vi "Main.vi"() -> ()   [LabVIEW 2020]
uses:
  Typedef/State.ctl
  Bundle Builder/Bundle Builder.lvclass
  Bundle Builder/Bundle Builder.lvclass/Bundle Builder.ctl
  bd79d48e-615b-41ab-9cb3-2d2f9496b7e1.vi
  Bundle Builder/Read Bundle Definition.vi
  Bundle Builder/Read Product Installers.vi
  Bundle Builder/Read Custom Actions.vi
  Bundle Builder/Read Element of Custom Actions Defnition.vi/bd8829dc-8fc1-4ce8-8fca-fa4916f1d24d.vi
  Bundle Builder/Read Element of Product Installers Definition.vi/92f76918-1563-4c6f-99b4-6a0cba476cd6.vi
  <vilib>/Comparison/Equal/Equal Functor/Equal Functor.lvclass
panel:
  in  "Clear Disk":bool
  in  "Stop Button":bool
  in  "Save":bool
  in  "Tab":T1(tab)
  in  "Bundle Definition":T2
  out "Product Key Unique?":bool
  in  "Product Installers":cluster{"Key":string, "Version":string}[](array[cluster])
  in  "Product Installer":T3 caption="NI Product Installer / Custom Product Installer"
  in  "Custom Actions":cluster{"Key":string, "Timing":string}[](array[cluster])
  out "Custom Action Key Unique?":bool
  in  "Custom Action":T4
  in  "Open":bool
  in  "Definitions":string(tree)
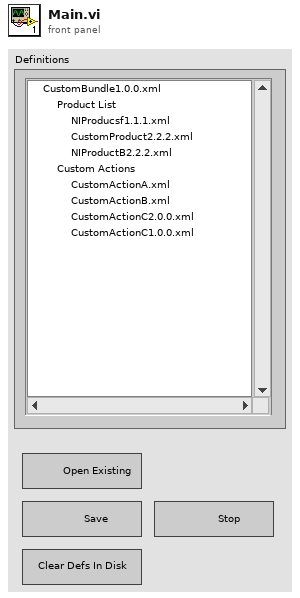
[diagram p1: front panel]
types:
  T1 = enum32{"Default", "Bundle", "Product List", "Product", "Custom Actions", "Custom Action"}
  T2 = cluster{"Key":string, "Display Name":string, "STS Software":string}
  T3 = cluster{"Display Name":string, "Type":enum16{"NI Installer", "Custom Installer"}, "Install Commands":cluster{"Path":string, "Parameters":string, "Successful Exit Codes":string, "Log Command":cluster{"Flag":string, "File Name":string}}[], "Uninstall Commands":cluster{"Path":string, "Parameters":string, "Successful Exit Codes":string, "Log Command":cluster{"Flag":string, "File Name":string}}[]}
  T4 = cluster{"Display Name":string, "Commands":cluster{"Path":string, "Parameters":string, "Successful Exit Codes":string}[]}
  T5 = typedef "State.ctl" = enum16{"Initialize", "Ready", "Open Bundle", "Show Selection Details"}
  T6 = enum8{"Enabled", "Disabled", "Disabled and Grayed Out"}
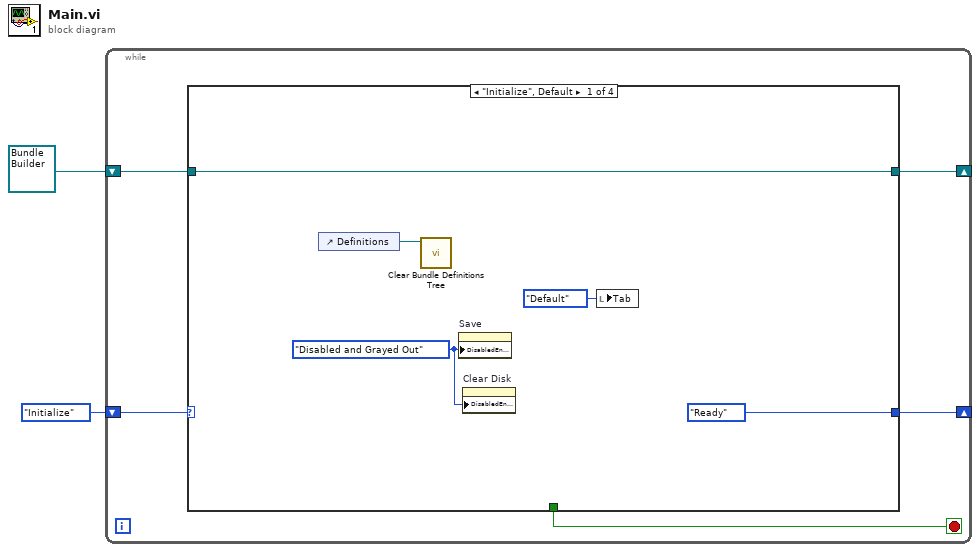
[diagram p0: block diagram]
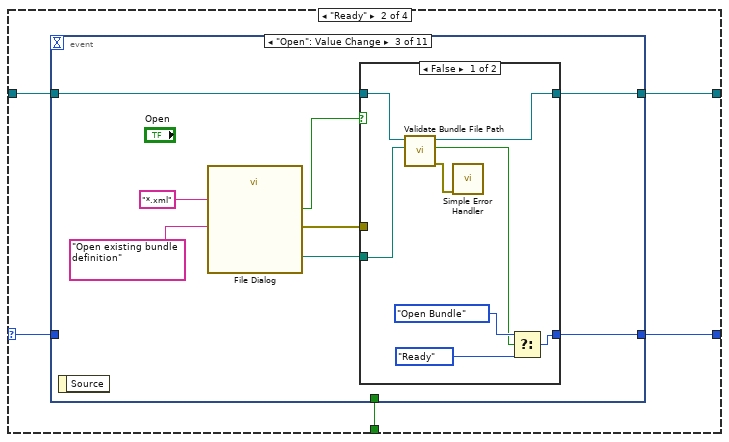
[diagram p2: hidden frame]
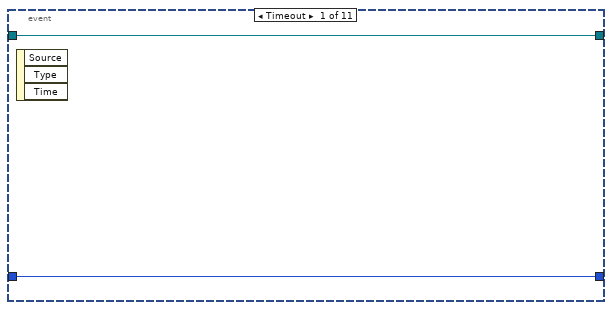
[diagram p3: hidden frame]
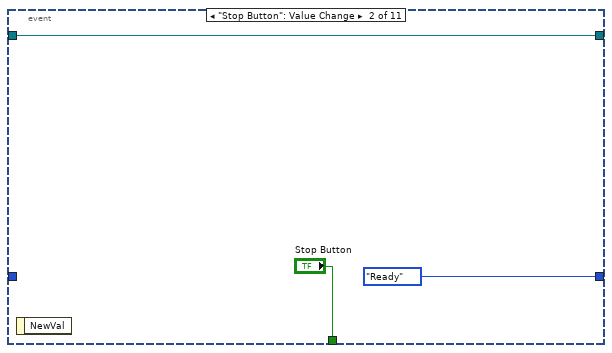
[diagram p4: hidden frame]
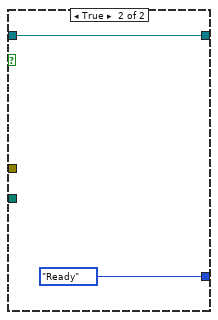
[diagram p5: hidden frame]
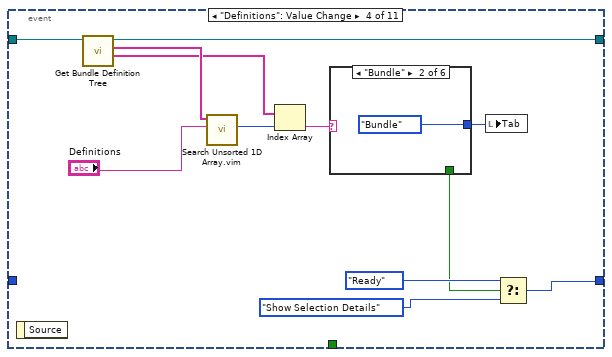
[diagram p6: hidden frame]
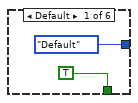
[diagram p7: hidden frame]
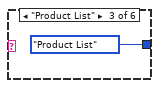
[diagram p8: hidden frame]
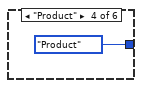
[diagram p9: hidden frame]
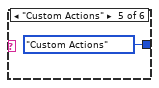
[diagram p10: hidden frame]
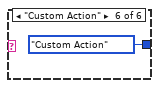
[diagram p11: hidden frame]
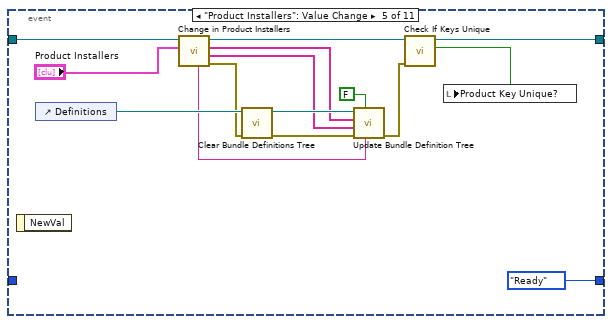
[diagram p12: hidden frame]
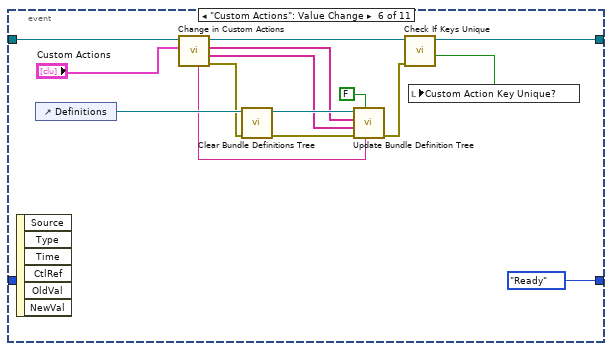
[diagram p13: hidden frame]
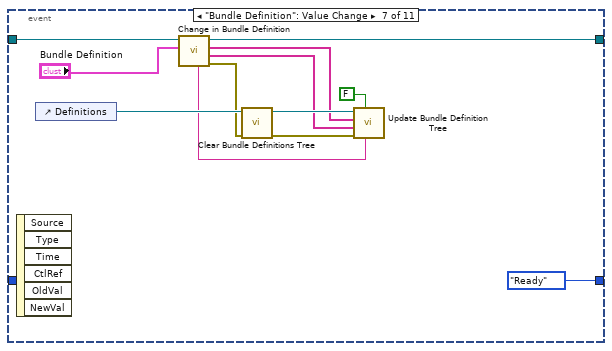
[diagram p14: hidden frame]
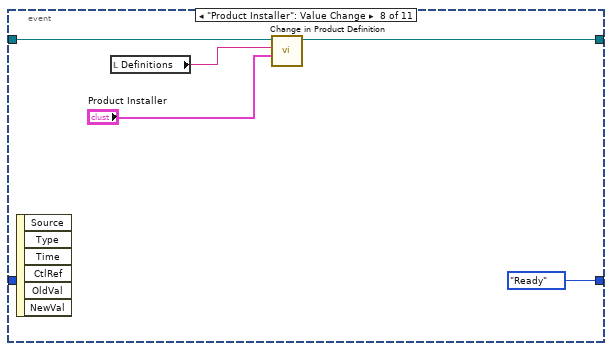
[diagram p15: hidden frame]
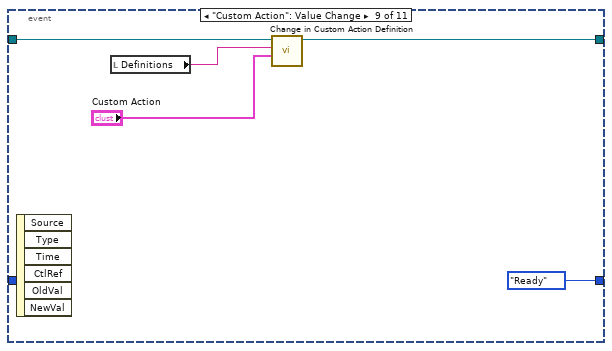
[diagram p16: hidden frame]
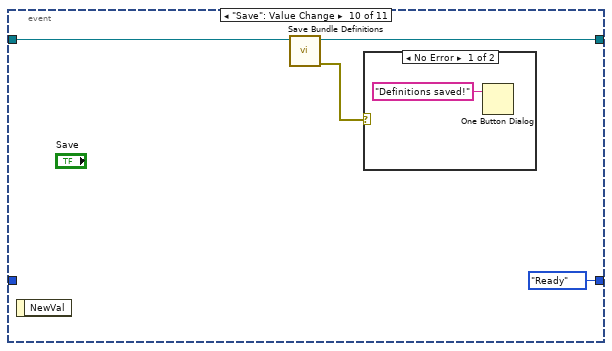
[diagram p17: hidden frame]
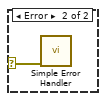
[diagram p18: hidden frame]
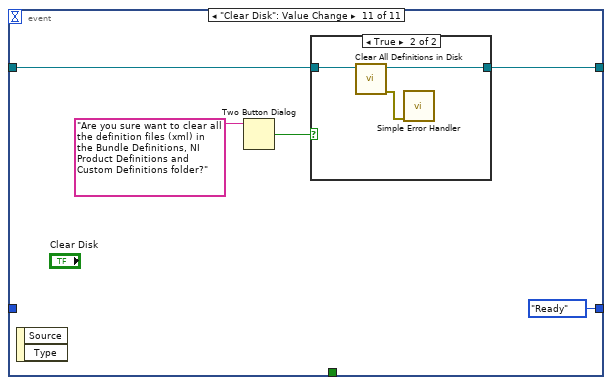
[diagram p19: hidden frame]
diagram:
  n1 = while {
    shift-right: [w3] -> _
    shift-left: State."Initialize" -> [w7]
    shift-right: [w4] -> _
    shift-left: refnum<class "Bundle Builder.lvclass"> refnum ("Bundle Builder.lvclass") -> [w5]
    stop <- w6 stop-if-true
    n2 = case shown="\"Initialize\", Default" w7 {
      selector: w7 -> [_ w14 _ _]
      tunnel: [_ w17 _ _] -> w6
      tunnel: w5 -> [w11 w16 w142 w147]
      tunnel: [w11 w15 w132 w146] -> w4
      tunnel: [State."Ready" w13 State."Ready" State."Ready"] -> w3
      frame "Initialize", Default {
        w8 = T6."Disabled and Grayed Out" ("Disabled")
        n3 = control-ref of="Definitions"() -> (w12:refnum<vi>)
        n4 = call "Clear Bundle Definitions Tree.vi"("TreeControl in"=w12) -> ()  [unwired: 9 in, 2 out]
        n5 = property on="Save" class="Bool"("DisabledEnum"=w8) -> ()  [unwired: 2 in, 2 out]
        n6 = property on="Clear Disk" class="Bool"("DisabledEnum"=w8) -> ()  [unwired: 2 in, 2 out]
        n7 = local write "Tab"(T1."Default" ("Tab")) -> ()
      }
      frame "Ready" {
        n8 = event shown="[2] \"Open\": Value Change" {
          selector: _ -> [_ _ _ _ _ _ _ _ _ _ _]
          dyn-events: _ -> [_ _ _ _ _ _ _ _ _ _ _]
          timeout: _ -> [_ _ _ _ _ _ _ _ _ _ _]
          tunnel: [_ "Stop Button" _ _ _ _ _ _ _ _ _] -> w17
          tunnel: [w18 State."Ready" w27 w43 State."Ready" State."Ready" State."Ready" State."Ready" State."Ready" State."Ready" State."Ready"] -> w13
          tunnel: w16 -> [w19 w20 w30 w52 w74 w89 w101 w106 w111 w115 w122]
          tunnel: [w19 w20 w29 w51 w62 w78 w98 w105 w110 w114 w120] -> w15
          tunnel: w14 -> [w18 _ _ _ _ _ _ _ _ _ _]
          event Timeout {
            n9 = event-data() -> ()  [unwired: 1 in, 3 out]
          }
          event "Stop Button": Value Change {
            n10 = event-data() -> ()  [unwired: 1 in, 1 out]
          }
          event "Open": Value Change {
            n11 = event-data() -> ()  [unwired: 1 in, 1 out]
            n12 = call "File Dialog"("prompt"="Open existing bundle definition", "pattern (all files)"="*.xml") -> ("selected path"=w26:path, "cancelled"=w28:bool, "error out"=w23:errorcluster)  [unwired: 10 in, 1 out]
            n13 = case shown="False" w28 {
              tunnel: w30 -> [w36 w40]
              tunnel: [w37 w40] -> w29
              tunnel: [w34 State."Ready"] -> w27
              tunnel: w26 -> [w35 _]
              tunnel: w23 -> [_ _]
              frame False {
                n14 = call "Validate Bundle File Path.vi"("Bundle File Path"=w35, "Bundle Builder in"=w36) -> ("error out"=w31:errorcluster, "Valid?"=w33:bool, "Bundle Builder out"=w37:refnum<class "Bundle Builder.lvclass">)  [unwired: 7 in]
                n15 = call <vilib>:"Simple Error Handler.vi"("error in (no error)"=w31) -> ()  [unwired: 4 in, 5 out]
                n16 = Select(t=State."Open Bundle", s=w33, f=State."Ready") -> (s? t:f=w34:T5)
              }
              frame True {
              }
            }
          }
          event "Definitions": Value Change {
            n17 = event-data() -> ()  [unwired: 1 in, 1 out]
            n18 = call "Get Bundle Definition Tree.vi"("Bundle Builder in"=w52) -> ("Tree Selection Types"=w48:string[], "Tree Selections"=w50:string[], "Bundle Builder out"=w51:refnum<class "Bundle Builder.lvclass">)  [unwired: 7 in, 1 out]
            n19 = call "Search Unsorted 1D Array.vim"("element"="Definitions", "unsorted 1D array"=w50) -> ("index of element"=w47:i32)  [unwired: 9 in]
            n20 = Index Array(array=w48, index=w47) -> (element=w46:string)
            n21 = case shown="\"Bundle\"" w46 {
              tunnel: [T1."Default" ("Tab") T1."Bundle" ("Tab") T1."Product List" ("Tab") T1."Product" ("Tab") T1."Custom Actions" ("Tab") T1."Custom Action" ("Tab")] -> w45
              tunnel: [TRUE _ _ _ _ _] -> w42
              frame Default {
              }
              frame "Bundle" {
              }
              frame "Product List" {
              }
              frame "Product" {
              }
              frame "Custom Actions" {
              }
              frame "Custom Action" {
              }
            }
            n22 = local write "Tab"(w45) -> ()
            n23 = Select(t=State."Ready", s=w42, f=State."Show Selection Details") -> (s? t:f=w43:T5)
          }
          event "Product Installers": Value Change {
            n24 = event-data() -> ()  [unwired: 1 in, 1 out]
            n25 = control-ref of="Definitions"() -> (w73:refnum<vi>)
            n26 = call "Change in Product Installers.vi"("Product Installers"="Product Installers", "Bundle Builder in"=w74) -> ("error out"=w65:errorcluster, "Custom Actions File Names"=w68:string[], "Product List File Names"=w69:string[], "Bundle Builder out"=w71:refnum<class "Bundle Builder.lvclass">, "Bundle Filename"=w67:string)  [unwired: 5 in]
            n27 = call "Clear Bundle Definitions Tree.vi"("error in"=w65, "TreeControl in"=w73) -> ("error out"=w66:errorcluster, "TreeControl out"=w72:refnum<vi>)  [unwired: 8 in]
            n28 = call "Update Bundle Definition Tree.vi"("Bundle Filename"=w67, "Reset Selection to Root? (T)"=FALSE, "error in"=w66, "Custom Actions File Names"=w68, "Product List File Names"=w69, "TreeControl in"=w72) -> ("error out"=w61:errorcluster)  [unwired: 4 in, 1 out]
            n29 = call "Check If Keys Unique.vi"("error in (no error)"=w61, "Bundle Builder in"=w71) -> ("Product Key Unique?"=w60:bool, "Bundle Builder out"=w62:refnum<class "Bundle Builder.lvclass">)  [unwired: 6 in, 2 out]
            n30 = local write "Product Key Unique?"(w60) -> ()
          }
          event "Custom Actions": Value Change {
            n31 = event-data() -> ()  [unwired: 1 in, 6 out]
            n32 = control-ref of="Definitions"() -> (w88:refnum<vi>)
            n33 = call "Change in Custom Actions.vi"("Custom Actions"="Custom Actions", "Bundle Builder in"=w89) -> ("error out"=w81:errorcluster, "Custom Actions File Names"=w84:string[], "Product List File Names"=w85:string[], "Bundle Builder out"=w86:refnum<class "Bundle Builder.lvclass">, "Bundle Filename"=w83:string)  [unwired: 5 in]
            n34 = call "Clear Bundle Definitions Tree.vi"("error in"=w81, "TreeControl in"=w88) -> ("error out"=w82:errorcluster, "TreeControl out"=w87:refnum<vi>)  [unwired: 8 in]
            n35 = call "Update Bundle Definition Tree.vi"("Bundle Filename"=w83, "Reset Selection to Root? (T)"=FALSE, "error in"=w82, "Custom Actions File Names"=w84, "Product List File Names"=w85, "TreeControl in"=w87) -> ("error out"=w77:errorcluster)  [unwired: 4 in, 1 out]
            n36 = call "Check If Keys Unique.vi"("error in (no error)"=w77, "Bundle Builder in"=w86) -> ("Custom Action Key Unique?"=w75:bool, "Bundle Builder out"=w78:refnum<class "Bundle Builder.lvclass">)  [unwired: 6 in, 2 out]
            n37 = local write "Custom Action Key Unique?"(w75) -> ()
          }
          event "Bundle Definition": Value Change {
            n38 = event-data() -> ()  [unwired: 1 in, 6 out]
            n39 = control-ref of="Definitions"() -> (w100:refnum<vi>)
            n40 = call "Change in Bundle Definition.vi"("Bundle Definition"="Bundle Definition", "Bundle Builder in"=w101) -> ("error out"=w93:errorcluster, "Custom Actions File Names"=w96:string[], "Product List File Names"=w97:string[], "Bundle Builder out"=w98:refnum<class "Bundle Builder.lvclass">, "Bundle Filename"=w95:string)  [unwired: 5 in]
            n41 = call "Clear Bundle Definitions Tree.vi"("error in"=w93, "TreeControl in"=w100) -> ("error out"=w94:errorcluster, "TreeControl out"=w99:refnum<vi>)  [unwired: 8 in]
            n42 = call "Update Bundle Definition Tree.vi"("Bundle Filename"=w95, "Reset Selection to Root? (T)"=FALSE, "error in"=w94, "Custom Actions File Names"=w96, "Product List File Names"=w97, "TreeControl in"=w99) -> ()  [unwired: 4 in, 2 out]
          }
          event "Product Installer": Value Change {
            n43 = event-data() -> ()  [unwired: 1 in, 6 out]
            n44 = local read "Definitions"() -> (w103:string)
            n45 = call "Change in Product Definition.vi"("Product Installer"="Product Installer", "Selected Product File Name"=w103, "Bundle Builder in"=w106) -> ("Bundle Builder out"=w105:refnum<class "Bundle Builder.lvclass">)  [unwired: 7 in, 1 out]
          }
          event "Custom Action": Value Change {
            n46 = event-data() -> ()  [unwired: 1 in, 6 out]
            n47 = local read "Definitions"() -> (w108:string)
            n48 = call "Change in Custom Action Definition.vi"("Custom Action"="Custom Action", "Selected Custom Action File Name"=w108, "Bundle Builder in"=w111) -> ("Bundle Builder out"=w110:refnum<class "Bundle Builder.lvclass">)  [unwired: 7 in, 1 out]
          }
          event "Save": Value Change {
            n49 = event-data() -> ()  [unwired: 1 in, 1 out]
            n50 = call "Save Bundle Definitions.vi"("Bundle Builder in"=w115) -> ("error out"=w113:errorcluster, "Bundle Builder out"=w114:refnum<class "Bundle Builder.lvclass">)  [unwired: 9 in]
            n51 = case shown="No Error" w113 {
              selector: w113 -> [_ w117]
              frame No Error {
                n52 = One Button Dialog(message="Definitions saved!") -> ()  [unwired: 1 in, 1 out]
              }
              frame Error {
                n53 = call <vilib>:"Simple Error Handler.vi"("error in (no error)"=w117) -> ()  [unwired: 4 in, 5 out]
              }
            }
          }
          event "Clear Disk": Value Change {
            n54 = event-data() -> ()  [unwired: 1 in, 2 out]
            n55 = Two Button Dialog(message="Are you sure want to clear all the definition files (xml) in the Bundle Definitions, NI Product Definitions and Custom Definitions folder?") -> (T button?=w119:bool)  [unwired: 2 in]
            n56 = case shown="True" w119 {
              tunnel: w122 -> [w123 w126]
              tunnel: [w123 w125] -> w120
              frame False {
              }
              frame True {
                n57 = call "Clear All Definitions in Disk.vi"("Bundle Builder in"=w126) -> ("error out"=w124:errorcluster, "Bundle Builder out"=w125:refnum<class "Bundle Builder.lvclass">)  [unwired: 9 in]
                n58 = call <vilib>:"Simple Error Handler.vi"("error in (no error)"=w124) -> ()  [unwired: 4 in, 5 out]
              }
            }
          }
        }
      }
      frame "Open Bundle" {
        w127 = T6."Enabled" ("Disabled")
        n59 = control-ref of="Definitions"() -> (w140:refnum<vi>)
        n60 = call "Open Bundle.vi"("Bundle Builder in"=w142) -> ("error out"=w134:errorcluster, "Custom Actions File Names"=w138:string[], "Product List File Names"=w139:string[], "Bundle Builder out"=w141:refnum<class "Bundle Builder.lvclass">, "Bundle Filename"=w137:string)  [unwired: 6 in]
        n61 = call "Clear Bundle Definitions Tree.vi"("error in"=w134, "TreeControl in"=w140) -> ("error out"=w133:errorcluster, "TreeControl out"=w135:refnum<vi>)  [unwired: 8 in]
        n62 = call "Update Bundle Definition Tree.vi"("Bundle Filename"=w137, "error in"=w133, "Custom Actions File Names"=w138, "Product List File Names"=w139, "TreeControl in"=w135) -> ("error out"=w131:errorcluster)  [unwired: 5 in, 1 out]
        n63 = call "Check If Keys Unique.vi"("error in (no error)"=w131, "Bundle Builder in"=w141) -> ("error out"=w128:errorcluster, "Custom Action Key Unique?"=→"Custom Action Key Unique?":bool, "Product Key Unique?"=→"Product Key Unique?":bool, "Bundle Builder out"=w132:refnum<class "Bundle Builder.lvclass">)  [unwired: 6 in]
        n64 = call <vilib>:"Simple Error Handler.vi"("error in (no error)"=w128) -> ()  [unwired: 4 in, 5 out]
        n65 = property on="Save" class="Bool"(error in=w128, "DisabledEnum"=w127) -> ()  [unwired: 1 in, 2 out]
        n66 = property on="Clear Disk" class="Bool"(error in=w128, "DisabledEnum"=w127) -> ()  [unwired: 1 in, 2 out]
      }
      frame "Show Selection Details" {
        n67 = local read "Definitions"() -> (w144:string)
        n68 = case shown="Default" "Tab" {
          tunnel: w147 -> [w148 w151 w154 w157 w161 w165]
          tunnel: [w148 w150 w153 w156 w160 w164] -> w146
          tunnel: w144 -> [_ _ _ _ w158 w162]
          frame Default {
          }
          frame "Bundle" {
            n69 = property class="Bundle Builder.lvclass"(reference=w151) -> (reference out=w150:refnum<class "Bundle Builder.lvclass">, "Bundle Definition"=w149:T2)  [unwired: 1 in, 1 out]
            n70 = local write "Bundle Definition"(w149) -> ()
          }
          frame "Product List" {
            n71 = property class="Bundle Builder.lvclass"(reference=w154) -> (reference out=w153:refnum<class "Bundle Builder.lvclass">, "Product Installers"=w152:cluster{"Key":string, "Version":string}[])  [unwired: 1 in, 1 out]
            n72 = local write "Product Installers"(w152) -> ()
          }
          frame "Custom Actions" {
            n73 = property class="Bundle Builder.lvclass"(reference=w157) -> (reference out=w156:refnum<class "Bundle Builder.lvclass">, "Custom Actions"=w155:cluster{"Key":string, "Timing":string}[])  [unwired: 1 in, 1 out]
            n74 = local write "Custom Actions"(w155) -> ()
          }
          frame "Custom Action" {
            n75 = call "Read Element of Custom Actions Defnition.vi"("Selected Custom Action File Name"=w158, "Bundle Builder in"=w161) -> ("Custom Actions"=w159:T4, "Bundle Builder out"=w160:refnum<class "Bundle Builder.lvclass">)  [unwired: 7 in, 1 out]
            n76 = local write "Custom Action"(w159) -> ()
          }
          frame "Product" {
            n77 = call "Read Element of Product Installers Definition.vi"("Selected Product File Name"=w162, "Bundle Builder in"=w165) -> ("Product Installer"=w163:T3, "Bundle Builder out"=w164:refnum<class "Bundle Builder.lvclass">)  [unwired: 7 in, 1 out]
            n78 = local write "Product Installer"(w163) -> ()
          }
        }
      }
    }
  }
